vi "Write Suggestion IO.vi"(8 "error in (no error)":errorcluster, 10 "Suggestion IO":refnum<class "SuggestionIObase.lvclass">, 11 "IntelliSenseStringControl in":refnum<class "IntelliSenseStringControl.lvclass">) -> (0 "error out":errorcluster, 3 "IntelliSenseStringControl out":refnum<class "IntelliSenseStringControl.lvclass">)   [LabVIEW 2016, in "StringIntelliSense.lvlib" / "IntelliSenseStringControl.lvclass"]
uses:
  IntelliSenseStringControl.lvclass
  Suggestions IO/base/SuggestionIObase.lvclass
  IntelliSenseStringControl.lvclass/IntelliSenseStringControl.ctl
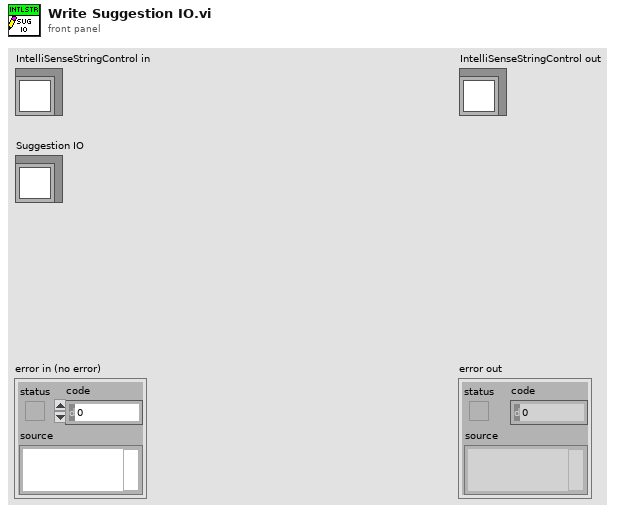
[diagram p1: front panel]
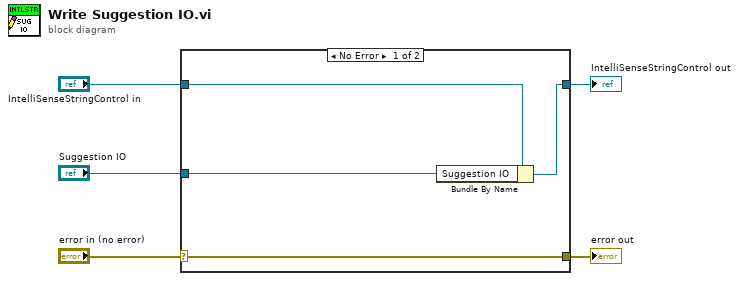
[diagram p0: block diagram]
diagram:
  n1 = case shown="No Error" "error in (no error)" {
    selector: "error in (no error)" -> [w9 w10]
    tunnel: [w9 w10] -> w4
    tunnel: [w7 w11] -> w2
    tunnel: "IntelliSenseStringControl in" -> [w8 w11]
    tunnel: "Suggestion IO" -> [w6 _]
    frame No Error {
      n2 = Bundle By Name(cluster=w8, "Suggestion IO"=w6) -> (w7:refnum<class "IntelliSenseStringControl.lvclass">)
    }
    frame Error {
    }
  }
  "error out" <- w4
  "IntelliSenseStringControl out" <- w2
